vi "getRandomColor.vi"() -> (0 "color":u32(colorbox))   [LabVIEW 2023]
uses:
  <vilib>/numeric/Random Number (Range) U64.vi
  <vilib>/numeric/sub_Random U32.vi
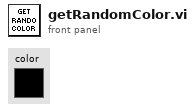
[diagram p1: front panel]
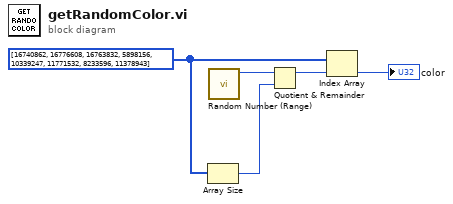
[diagram p0: block diagram]
diagram:
  w3 = u32[] [16740862, 16776608, 16763832, 5898156, 10339247, 11771532, 8233596, 11378943]
  n1 = Array Size(array=w3) -> (size(s)=w2:i32)
  n2 = call-poly <vilib>:"Random Number (Range).vi"() -> ("number"=w1:u64)  [unwired: 11 in]
  n3 = Quotient & Remainder(x=w1, y=w2) -> (x-y*floor(x/y)=w4:u64)  [unwired: 1 out]
  n4 = Index Array(array=w3, index=w4) -> (element=→"color":u32)
